vi "timed_event_to_file.vi"(8 "file error in":errorcluster, 10 "String":string, 11 "file ref in":refnum<file>) -> (0 "file error out":errorcluster, 3 "file ref out":refnum<file>)   [LabVIEW 2010]
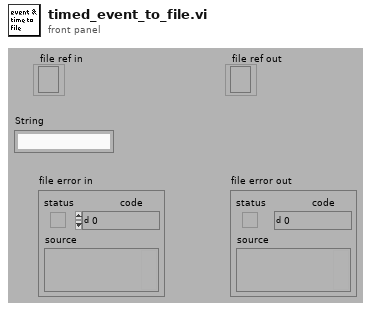
[diagram p1: front panel]
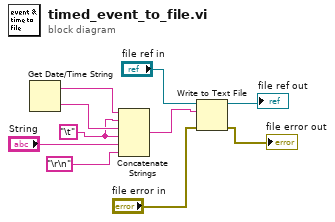
[diagram p0: block diagram]
diagram:
  w1 = "\t"
  n1 = Get Date/Time String() -> (date string=w2:string, time string=w3:string)  [unwired: 3 in]
  n2 = Concatenate Strings(w2, w1, w3, w1, "String", "\r\n") -> (w6:string)
  n3 = Write to Text File(file (use dialog)="file ref in", text=w6, error in="file error in") -> (refnum out=→"file ref out":refnum<file>, error out=→"file error out":errorcluster)  [unwired: 1 in, 1 out]
